vi "graph_redef_bounds.vi"(7 "reference":refnum<vi>, 8 "error in":errorcluster, 11 "graph refs in":refnum<vi>[](array[refnum])) -> (0 "error out":errorcluster, 3 "graph refs out":refnum<vi>[](array[refnum]))   [LabVIEW 2020]
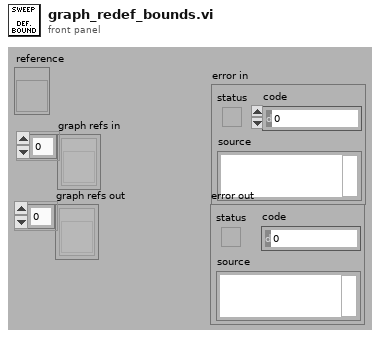
[diagram p1: front panel]
types:
  T1 = typedef "LVRectTypeDef.ctl" = cluster{"Left":i16, "Top":i16, "Right":i16, "Bottom":i16}
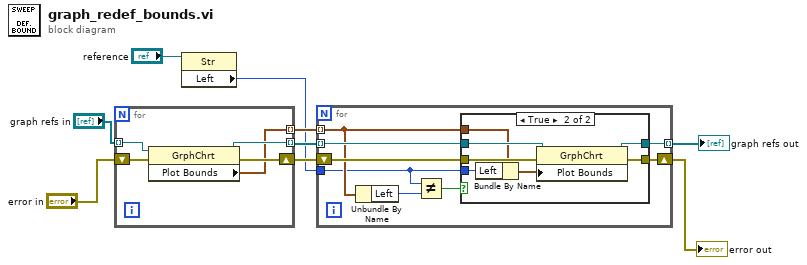
[diagram p0: block diagram]
diagram:
  n1 = for {
    tunnel: "graph refs in" -> [w14] mode=indexing
    tunnel: [w13] -> w9 mode=indexing
    shift-right: [w11] -> w8
    shift-left: "error in" -> [w12]
    tunnel: [w10] -> w7 mode=indexing
    n2 = property class="GrphChrt"(reference=w14, error in=w12) -> (reference out=w13:refnum<vi>, error out=w11:errorcluster, "Plot Bounds"=w10:T1)
  }
  n3 = property class="Str"(reference="reference") -> ("Left"=w4:i32)  [unwired: 1 in, 2 out]
  n4 = for {
    tunnel: w9 -> [w22] mode=indexing
    tunnel: [w21] -> w2 mode=indexing
    shift-right: [w19] -> w5
    shift-left: w8 -> [w20]
    tunnel: w7 -> [w18] mode=indexing
    tunnel: w4 -> [w16]
    n5 = Unbundle By Name(w18) -> ("Left"=w17:i16)
    n6 = Not Equal?(x=w16, y=w17) -> (x != y?=w15:bool)
    n7 = case shown="True" w15 {
      tunnel: w22 -> [w23 w31]
      tunnel: [w23 w30] -> w21
      tunnel: w20 -> [w24 w29]
      tunnel: [w24 w28] -> w19
      tunnel: w18 -> [_ w26]
      tunnel: w16 -> [_ w25]
      frame False {
      }
      frame True {
        n8 = Bundle By Name(cluster=w26, "Left"=w25) -> (w27:T1)
        n9 = property class="GrphChrt"(reference=w31, error in=w29, "Plot Bounds"=w27) -> (reference out=w30:refnum<vi>, error out=w28:errorcluster)
      }
    }
  }
  "error out" <- w5
  "graph refs out" <- w2
